vi "DS_GT_FileNames_To_MVTec_Format.vi"() -> ()   [LabVIEW 2020]
panel:
  out "error out":errorcluster
  in  "Folder Path":path=path "D:/DNN/_from_Customer/2024_04_19_Ayan_Ghosh_Capsule_Anomaly/2024_04_19/1_Datasets/13_Orig_Reduce_Train_200_Val_200/ground_truth/bad - Copy"
  out "Progress":i32
  out "Filenames":path[](array[path])
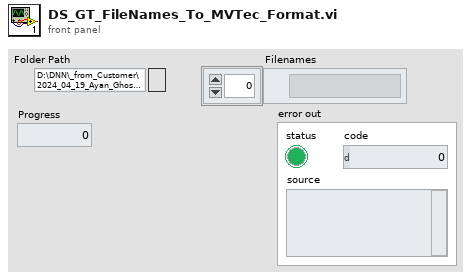
[diagram p1: front panel]
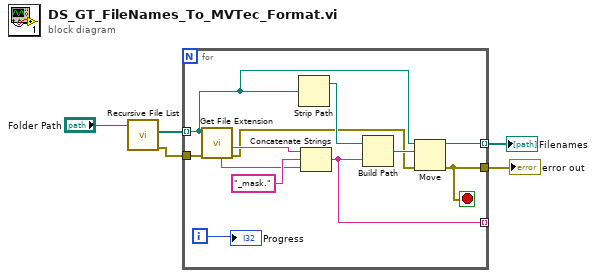
[diagram p0: block diagram]
diagram:
  n1 = call <vilib>:"Recursive File List.vi"("Folder Path"="Folder Path") -> ("error out"=w2:errorcluster, "All Files in Dir"=w5:path[])  [unwired: 6 in, 3 out]
  n2 = for {
    tunnel: w5 -> [w9] mode=indexing
    tunnel: [w13] -> _ mode=indexing
    tunnel: [w12] -> w3 mode=indexing
    tunnel: w2 -> [w8]
    tunnel: [w6] -> w1
    i -> [w11]
    stop <- w6 stop-if-true
    n3 = call <vilib>:"Get File Extension.vi"("error in (no error)"=w8, "file"=w9) -> ("error out"=w7:errorcluster, "filename without extension"=w17:string, "unmodified file extension"=w15:string)  [unwired: 5 in, 2 out]
    n4 = Strip Path(path=w9) -> (stripped path=w14:path)  [unwired: 1 out]
    n5 = Concatenate Strings(w17, "_mask." ("string"), w15) -> (w13:string)
    n6 = Build Path(base path=w14, name or relative path=w13) -> (appended path=w10:path)
    n7 = Move(source path=w9, error in=w7, 10:w10) -> (error out=w6:errorcluster, 3:w12:path)  [unwired: 2 in, 1 out]
    "Progress" <- w11
  }
  "Filenames" <- w3
  "error out" <- w1
